vi "BattlesonEXCtsk#5.vi"() -> ()   [LabVIEW 2014, in "Battleson_Robot_12-2-16.lvrbt"]
uses:
  C:/Users/blb1094/Documents/LabVIEW Data/NXTRobotics/Projects/Battleson_Robot_12-2-16/Battleson_Robot_12-2-16.lvrbt
  <vilib>/NXT/Dual Mode Library/Sensors/EV3_Ultrasonic_CM.vi
panel:
  in  "stop":bool
  out "Error?":bool
  out "wall proximity":string
  out "distance LED":bool
  out "current distance":dbl
  in  "min distance":sgl
  in  "max distance":sgl
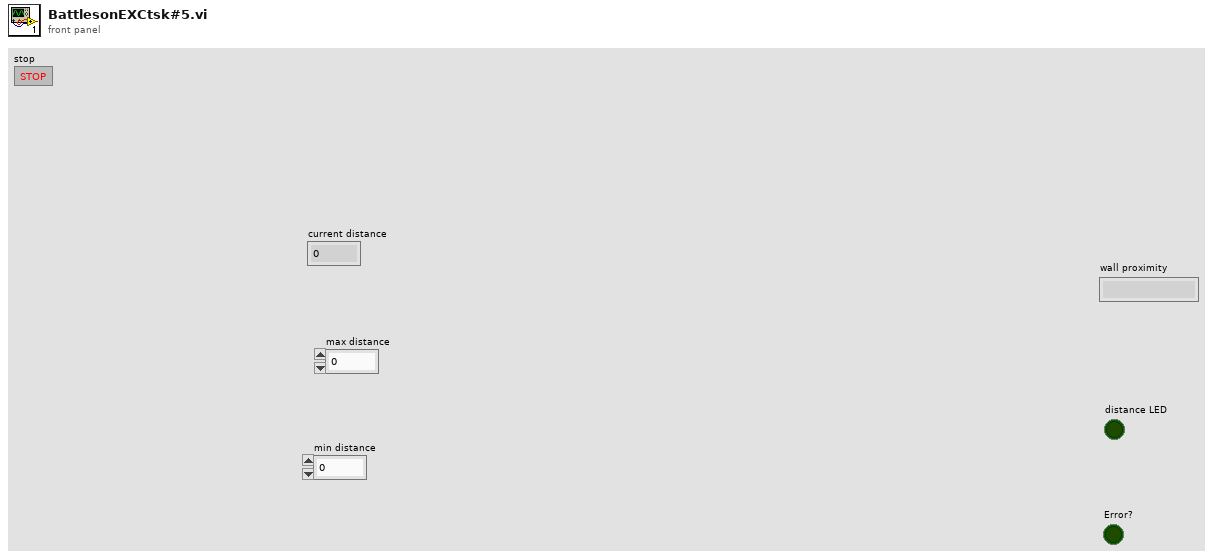
[diagram p1: front panel]
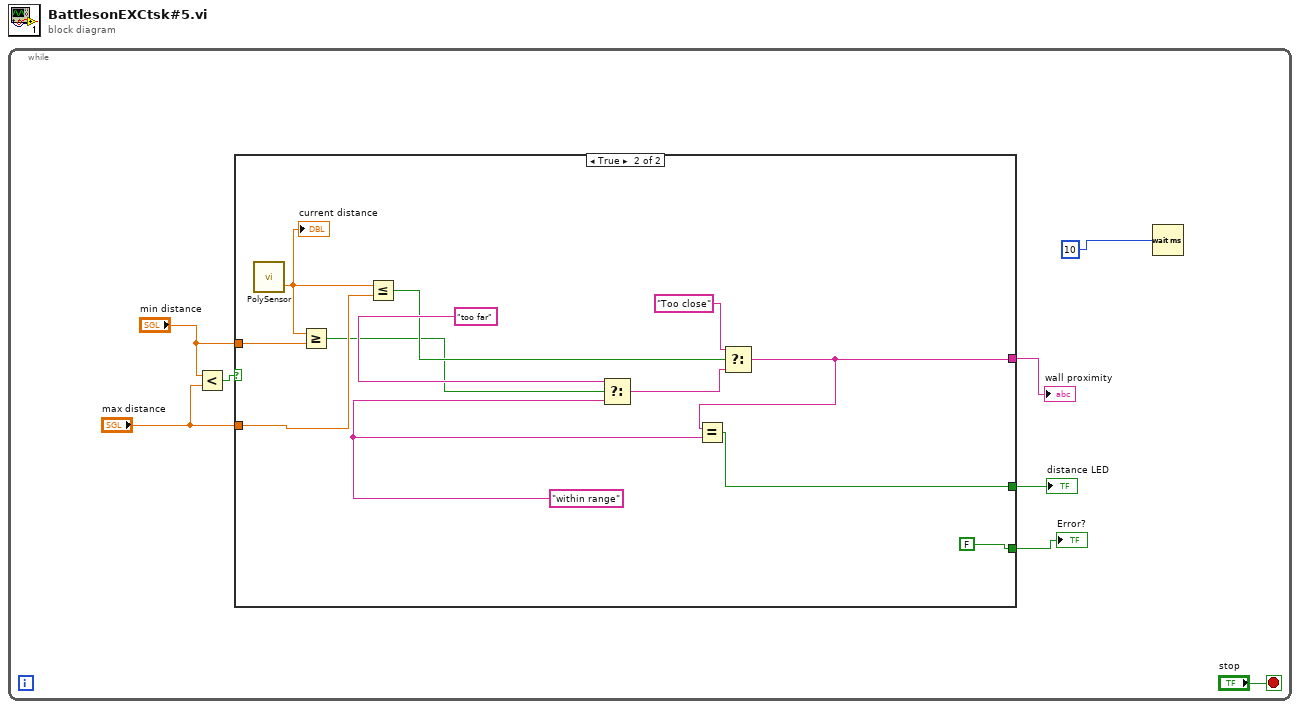
[diagram p0: block diagram]
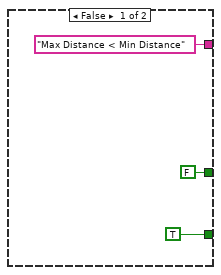
[diagram p2: hidden frame]
diagram:
  n1 = while {
    stop <- "stop" stop-if-true
    n2 = Less?(x="min distance", y="max distance") -> (x < y?=w3:bool)
    n3 = case shown="True" w3 {
      tunnel: "min distance" -> [_ w22]
      tunnel: "max distance" -> [_ w18]
      tunnel: [FALSE w17] -> w8
      tunnel: ["Max Distance < Min Distance" w13] -> w7
      tunnel: [TRUE FALSE] -> w1
      frame False {
      }
      frame True {
        w19 = "within range"
        n4 = call-poly <vilib>:"PolySensor.vi"() -> ("Centimeters"=w23:sgl)  [unwired: 3 in, 1 out]
        "current distance" <- w23
        n5 = Greater Or Equal?(x=w23, y=w22) -> (x >= y?=w16:bool)
        n6 = Less Or Equal?(x=w23, y=w18) -> (x <= y?=w20:bool)
        n7 = Select(t="too far", s=w16, f=w19) -> (s? t:f=w14:string)
        n8 = Select(t="Too close", s=w20, f=w14) -> (s? t:f=w13:string)
        n9 = Equal?(x=w13, y=w19) -> (x = y?=w17:bool)
      }
    }
    "distance LED" <- w8
    "wall proximity" <- w7
    "Error?" <- w1
    n10 = Wait (ms)(milliseconds to wait=u32 10) -> ()  [unwired: 1 out]
  }
